vi "SQLExecDirect.vi"(4 "error in (no error)":errorcluster, 6 "StatementText":string, 7 "InputHandle":i32) -> (0 "error out":errorcluster, 3 "OutputHandle":i32)   [LabVIEW 2011]
doc: "Execute entièrement la requête spécifiée par le lien"
uses:
  Odbc32.dll
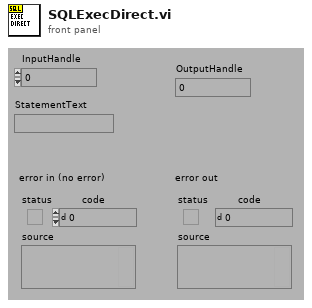
[diagram p1: front panel]
types:
  T1 = enum16{"NOPE", "SQL_HANDLE_ENV", "SQL_HANDLE_DBC", "SQL_HANDLE_STMT", "SQL_HANDLE_DESC"}
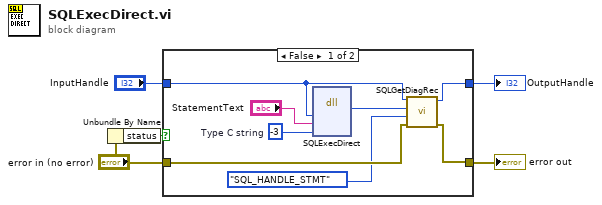
[diagram p0: block diagram]
diagram:
  n1 = Unbundle By Name("error in (no error)") -> ("status"=w4:bool)
  n2 = case shown="False" w4 {
    tunnel: "InputHandle" -> [w8 w14]
    tunnel: [w10 w15] -> w3
    tunnel: "error in (no error)" -> [w11 w15]
    tunnel: [w7 w14] -> w1
    frame False {
      w12 = -3  # Type C string
      n3 = dll-call lib="Odbc32.dll" fn="SQLExecDirect"("StatementHandle"=w8, "StatementText"="StatementText", "TextLength"=w12) -> (w9:i16)  [unwired: 6 in, 2 out]
      n4 = call "SQLGetDiagRec.vi"("error in (no error)"=w11, "HandleType"=T1."SQL_HANDLE_STMT", "Status (SQL_SUCCESS=0)"=w9, "Input Handle"=w8) -> ("error out"=w10:errorcluster, "Output Handle"=w7:i32)  [unwired: 2 out]
    }
    frame True {
    }
  }
  "OutputHandle" <- w1
  "error out" <- w3
